vi "Measurement Logic.vi"(8 "error in":errorcluster, 10 "Measurement Context":refnum<class "MeasurementContext.lvclass">, 11 "Measurement Configuration":T2={"Load Current in A"=0.005, "Nominal Output Voltage in V"=3.3, "Start"=4.0, "Stop"=6.0, "Step"=0.1, "Input SMU"="", "Load SMU"="", "Input DMM"="", "Load DMM"=""} {"Nominal Output Voltage in V" format="%#_13g"; "Load Current in A" format="%#_13g"}) -> (0 "error out":errorcluster, 2 "Measurement Context out":refnum<class "MeasurementContext.lvclass">, 3 "Measurement Results":T1)   [LabVIEW 2020, in "LineRegulation.lvlib"]
uses:
  LineRegulation.lvlib
  Measurement Configuration.ctl
  Measurement Results.ctl
  RPC Service/MeasurementContext/MeasurementContext.lvclass
  TestInputs.ctl
  Reusables/Advanced Settings.ctl
  Reusables/Prepare Fn Configurations.ctl
  Reusables/Load Output Function.ctl
  Reusables/Stimulus And Measure.ctl
  TestResults.ctl
  334814aa-6350-40fc-9da7-130e073bd573.vi
panel:
  out "Line Regulation":cluster{"Iload (mA)":dbl[], "Vout (V)":dbl[]}(graph)
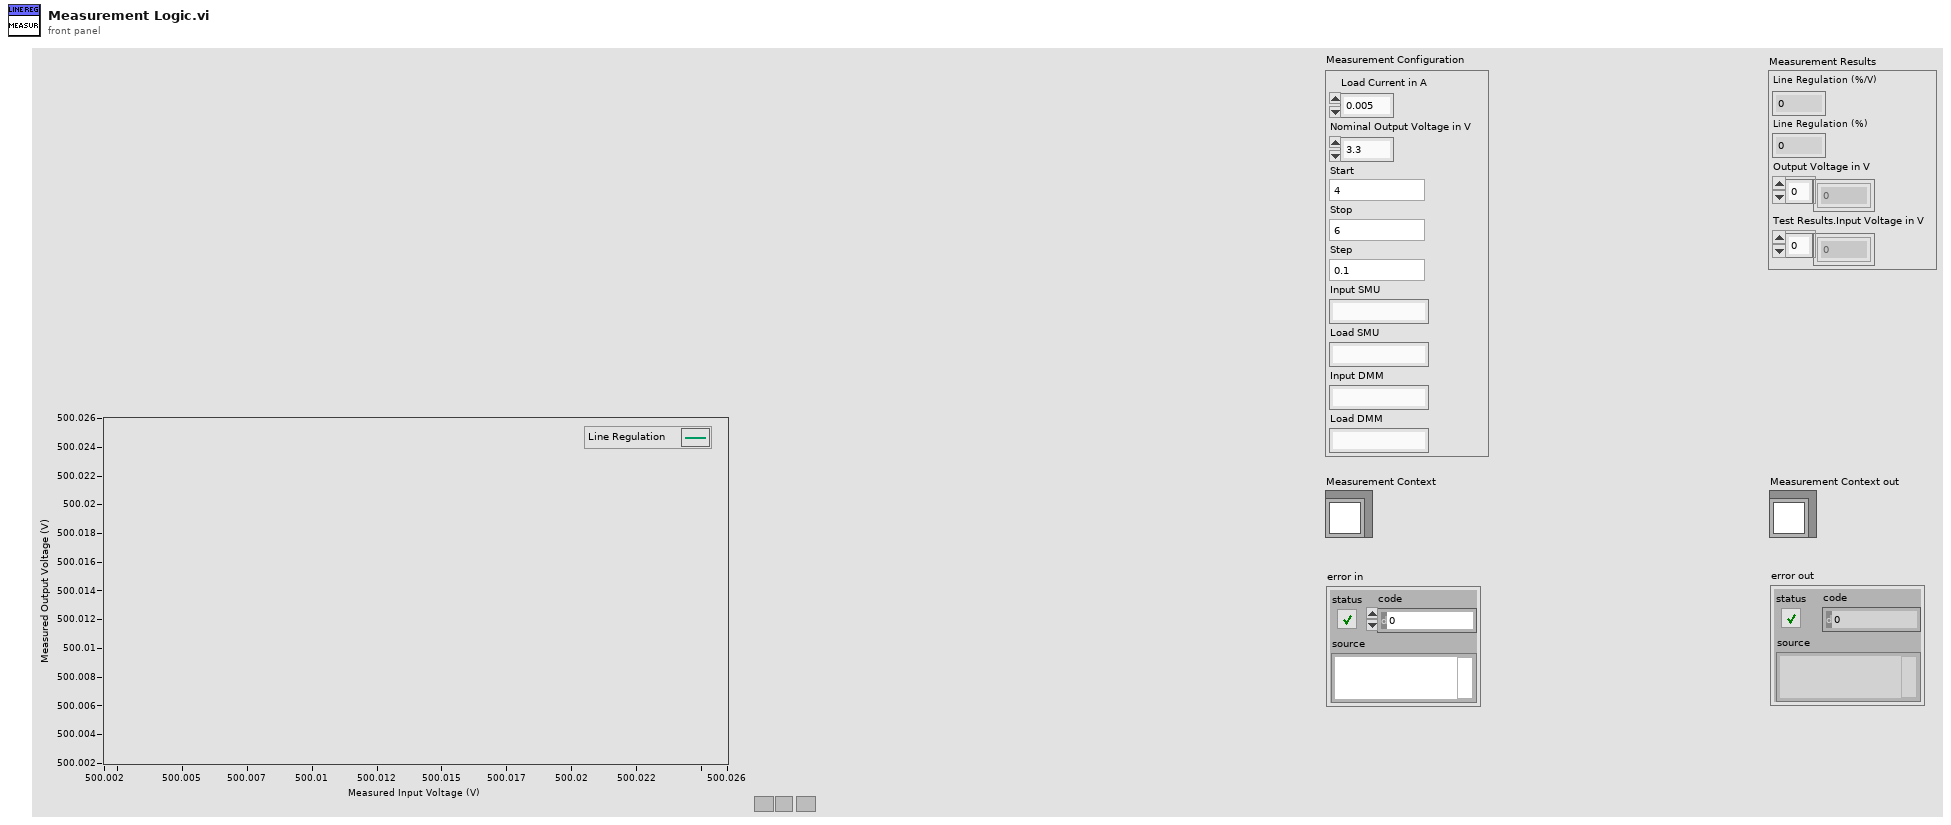
[diagram p1: front panel]
types:
  T1 = typedef "LineRegulation.lvlib/Measurement Results.ctl" = cluster{"Line Regulation (%/V)":dbl, "Line Regulation (%)":dbl, "Output Voltage in V":dbl[], "Test Results.Input Voltage in V":dbl[]}
  T2 = typedef "LineRegulation.lvlib/Measurement Configuration.ctl" = cluster{"Load Current in A":dbl, "Nominal Output Voltage in V":dbl, "Start":dbl, "Stop":dbl, "Step":dbl, "Input SMU":string, "Load SMU":string, "Input DMM":string, "Load DMM":string}
  T3 = typedef "LineRegulation.lvlib/TestInputs.ctl" = cluster{"Load Current in A":dbl, "Input Voltage in V":dbl[], "Nominal Output Voltage in V":dbl, "Advance Setting":T4}
  T4 = typedef "Advanced Settings.ctl" = cluster{"Prepare":T5, "Stimulus And Measure":T7}
  T5 = typedef "Prepare Fn Configurations.ctl" = cluster{"Load SMU Output Function":T6}
  T6 = typedef "Load Output Function.ctl" = enum16{"VoltageSource", "CurrentSource"}
  T7 = typedef "Stimulus And Measure.ctl" = cluster{"Loop Delay in milliSecond":u32}
  T8 = typedef "LineRegulation.lvlib/TestResults.ctl" = cluster{"Input Voltage in V":dbl[], "Input Current in A":dbl[], "Output Voltage in V":dbl[], "Load Current in A":dbl[], "Line Regulation in %/V":dbl, "Line Regulation in %":dbl}
  T9 = cluster{"Test Inputs":T3, "Test Results":T8, "Test Results[][]":string[][], "SMU V":refnum<k15>, "Input DMM":refnum<k15>, "Load DMM":refnum<k15>, "SMU I":refnum<k15>}
  T10 = cluster{"Input Voltage in V":dbl[], "Output Voltage in V":dbl[]}
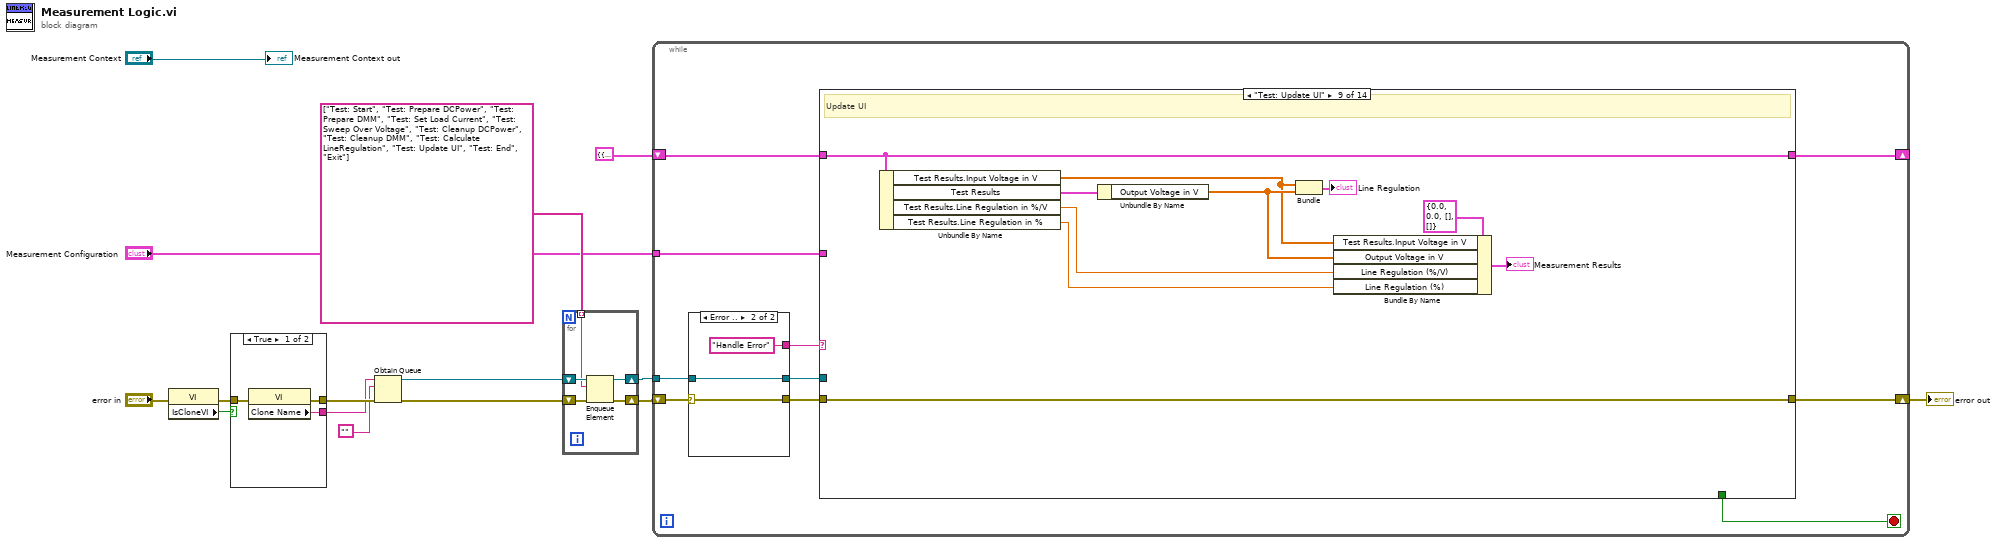
[diagram p0: block diagram]
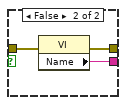
[diagram p2: hidden frame]
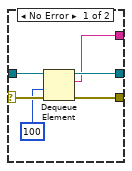
[diagram p3: hidden frame]
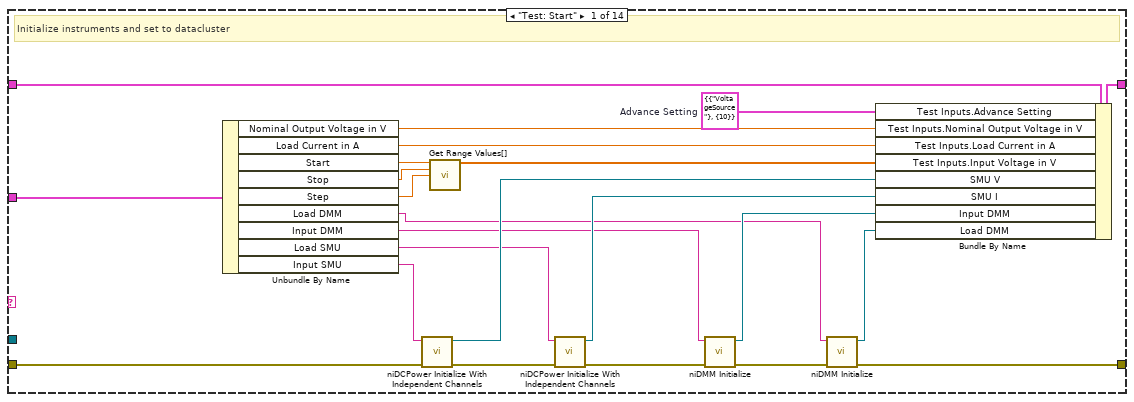
[diagram p4: hidden frame]
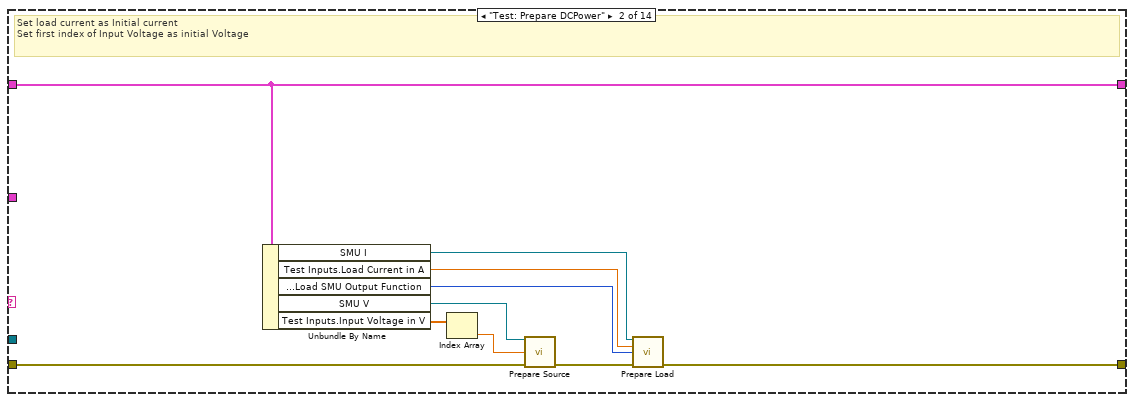
[diagram p5: hidden frame]
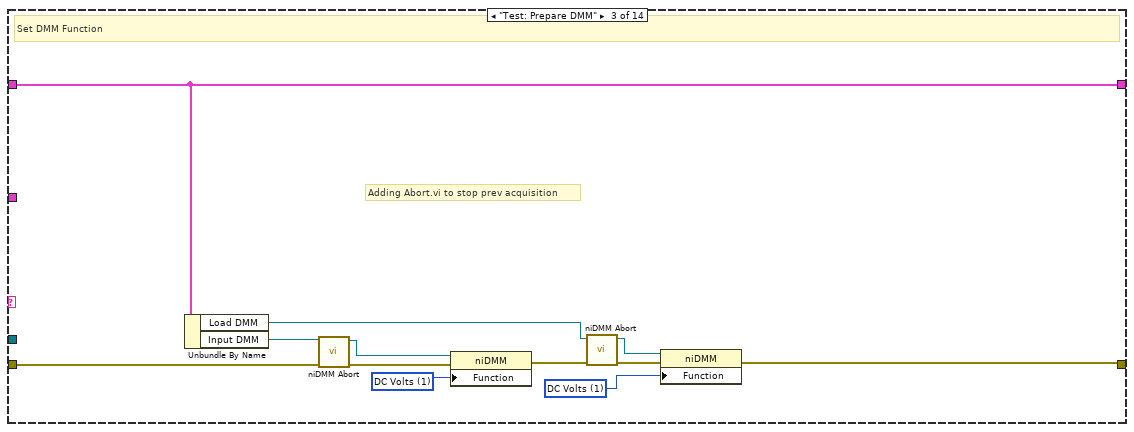
[diagram p6: hidden frame]
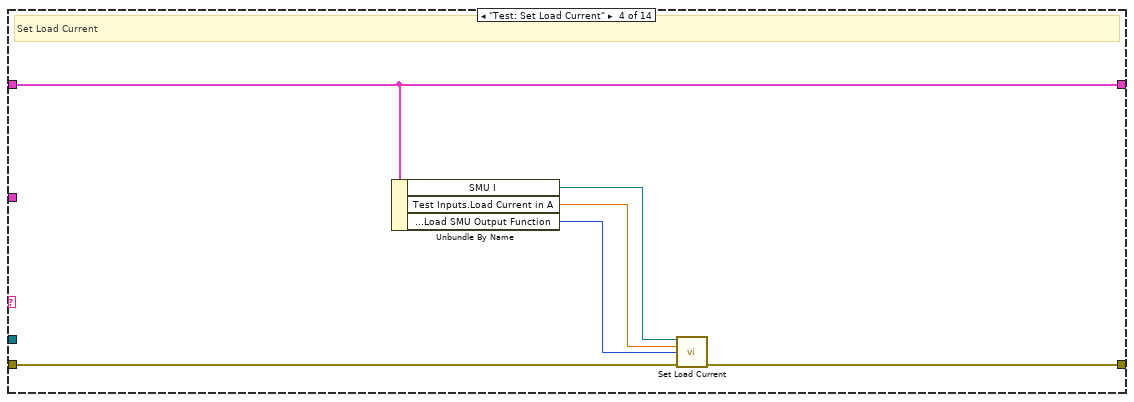
[diagram p7: hidden frame]
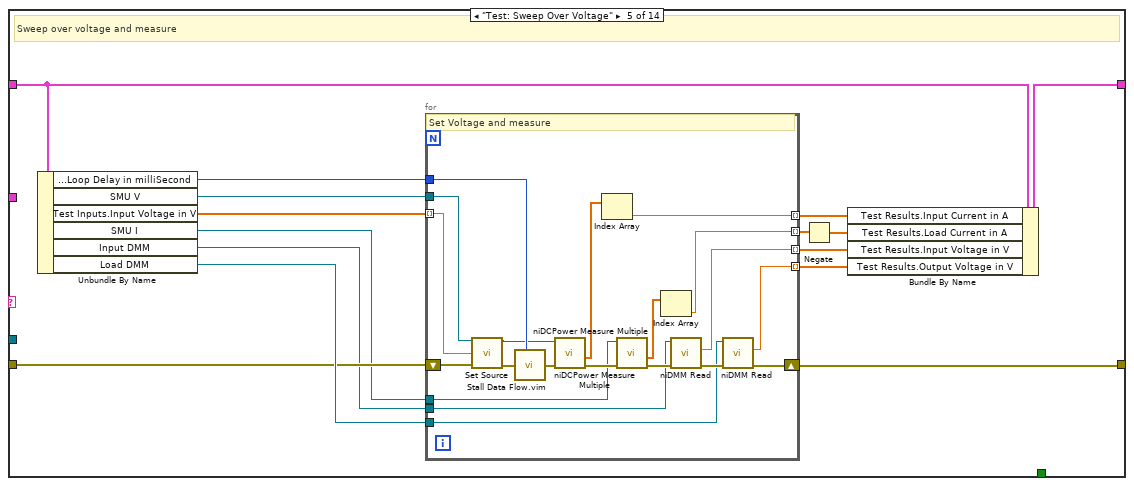
[diagram p8: hidden frame]
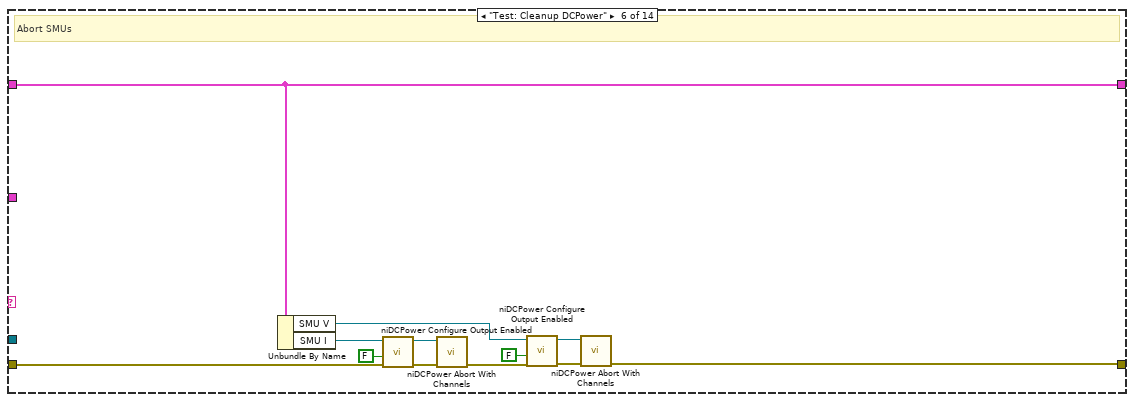
[diagram p9: hidden frame]
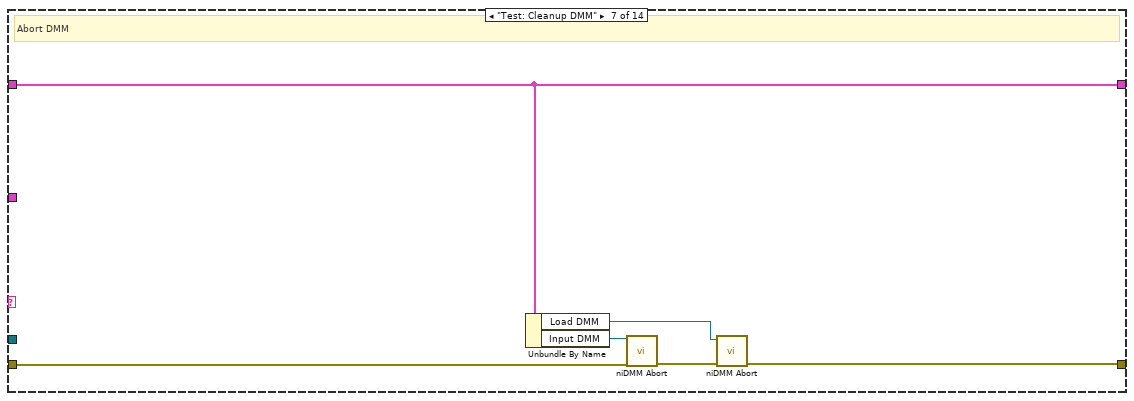
[diagram p10: hidden frame]
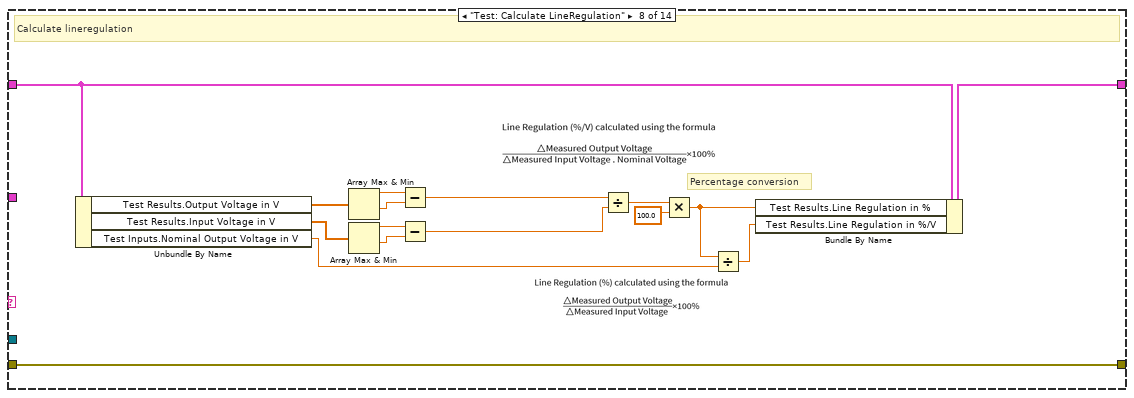
[diagram p11: hidden frame]
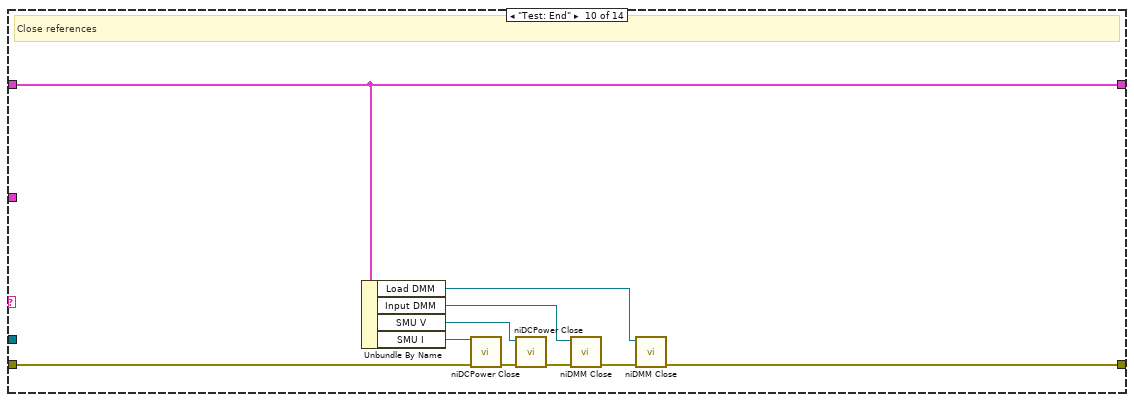
[diagram p12: hidden frame]
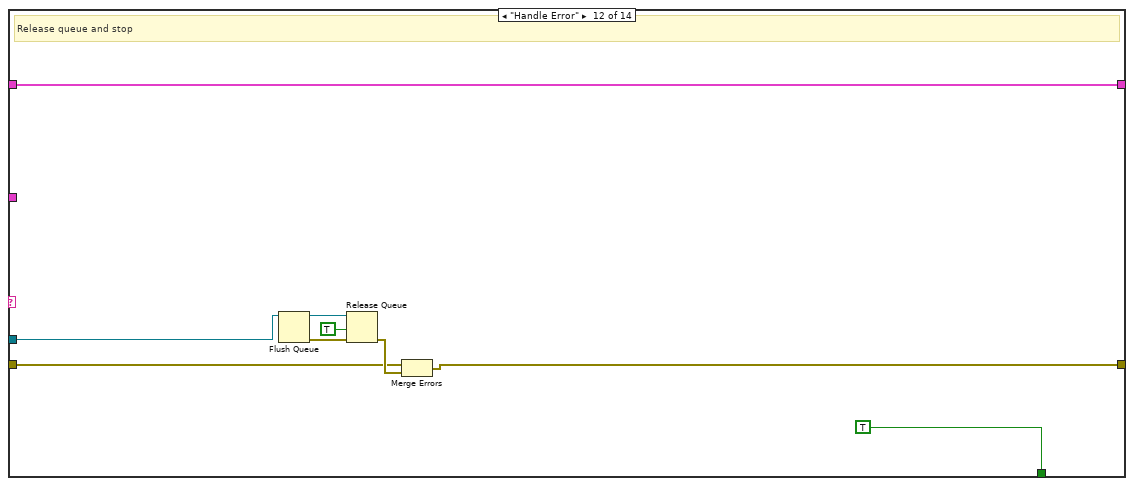
[diagram p14: hidden frame]
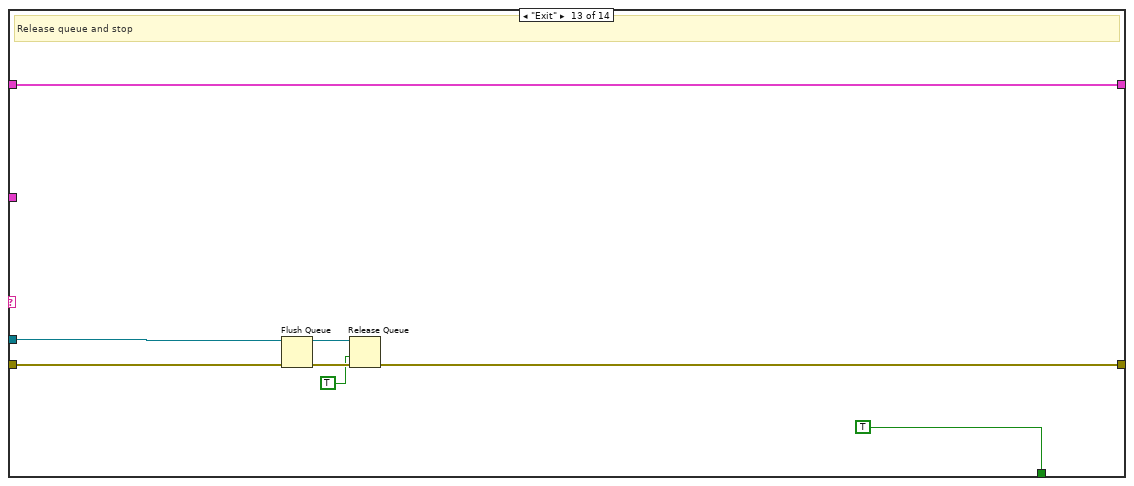
[diagram p15: hidden frame]
diagram:
  n1 = property class="VI"(error in="error in") -> (error out=w8:errorcluster, "IsCloneVI"=w9:bool)  [unwired: 1 in, 1 out]
  n2 = case shown="True" w9 {
    tunnel: [w18 w21] -> w14
    tunnel: [w17 w20] -> w13
    tunnel: w8 -> [w16 w19]
    frame True {
      n3 = property class="VI"(error in=w16) -> (error out=w18:errorcluster, "Clone Name"=w17:string)  [unwired: 1 in, 1 out]
    }
    frame False {
      n4 = property class="VI"(error in=w19) -> (error out=w21:errorcluster, "Name"=w20:string)  [unwired: 1 in, 1 out]
    }
  }
  n5 = Obtain Queue(name (unnamed)=w13, element data type="", error in (no error)=w14) -> (queue out=w11:refnum<queue>, error out=w12:errorcluster)  [unwired: 2 in, 1 out]
  n6 = for {
    shift-right: [w24] -> w7
    shift-left: w12 -> [w26]
    shift-right: [w23] -> w6
    shift-left: w11 -> [w25]
    tunnel: string[] ["Test: Start", "Test: Prepare DCPower", "Test: Prepare DMM", "Test: Set Load Current", "Test: Sweep Over Voltage", "Test: Cleanup DCPower", "Test: Cleanup DMM", "Test: Calculate LineRegulation", "Test: Update UI", "Test: End", "Exit"] -> [w22] mode=indexing
    n7 = Enqueue Element(queue=w25, element=w22, error in (no error)=w26) -> (queue out=w23:refnum<queue>, error out=w24:errorcluster)  [unwired: 1 in, 1 out]
  }
  n8 = while {
    shift-right: [w36] -> w2
    shift-left: w7 -> [w32]
    shift-right: [w34] -> _
    shift-left: T9 {"Test Inputs"={"Load Current in A"=0.0, "Input Voltage in V"=[], "Nominal Output Voltage in V"=0.0, "Advance Setting"={"Prepare"={"Load SMU Output Function"=enum."VoltageSource"}, "Stimulus And Measure"={"Loop Delay in milliSecond"=1}}}, "Test Results"={"Input Voltage in V"=[], "Input Current in A"=[], "Output Voltage in V"=[], "Load Current in A"=[], "Line Regulation in %/V"=0.0, "Line Regulation in %"=0.0}, "Test Results[][]"=[], "SMU V"="", "Input DMM"="", "Load DMM"="", "SMU I"=""} -> [w35]
    tunnel: w6 -> [w28]
    tunnel: "Measurement Configuration" -> [w27]
    stop <- w33 stop-if-true
    n9 = case shown="Error .." w32 {
      selector: w32 -> [w42 w45]
      tunnel: [w41 w45] -> w29
      tunnel: w28 -> [w40 w44]
      tunnel: [w39 w44] -> w31
      tunnel: [w38 "Handle Error"] -> w30
      frame No Error {
        n10 = Dequeue Element(queue=w40, timeout in ms (-1)=100, error in (no error)=w42) -> (queue out=w39:refnum<queue>, element=w38:string, error out=w41:errorcluster)  [unwired: 1 out]
      }
      frame Error {
      }
    }
    n11 = case shown="\"Test: Update UI\"" w30 {
      tunnel: w31 -> [_ _ _ _ _ _ _ _ _ _ _ w190 w197 _]
      tunnel: w29 -> [w51 w71 w79 w93 w99 w132 w144 w150 w168 w176 w187 w188 w199 w205]
      tunnel: [w50 w72 w81 w94 w102 w140 w147 w150 w168 w179 w187 w195 w198 w205] -> w36
      tunnel: w35 -> [w67 w77 w87 w96 w100 w139 w149 w151 w173 w185 w186 w196 w204 w206]
      tunnel: [w68 w77 w87 w96 w101 w139 w149 w152 w173 w185 w186 w196 w204 w206] -> w34
      tunnel: [_ _ _ _ _ _ _ _ _ _ _ TRUE TRUE _] -> w33
      tunnel: w27 -> [w46 _ _ _ _ _ _ _ _ _ _ _ _ _]
      frame "Test: Start" {
        w47 = T4 {"Prepare"={"Load SMU Output Function"=enum."VoltageSource"}, "Stimulus And Measure"={"Loop Delay in milliSecond"=10}}  # Advance Setting
        # "Initialize instruments and set to datacluster"
        n12 = Unbundle By Name(w46) -> ("Nominal Output Voltage in V"=w49:dbl, "Load Current in A"=w48:dbl, "Start"=w59:dbl, "Stop"=w58:dbl, "Step"=w57:dbl, "Load DMM"=w55:string, "Input DMM"=w54:string, "Load SMU"=w53:string, "Input SMU"=w52:string)
        n13 = call <instrlib>:"niDCPower Initialize With Independent Channels.vi"("error in (no error)"=w51, "resource name"=w52) -> ("error out"=w63:errorcluster, "instrument handle out"=w66:refnum<k15>)  [unwired: 8 in]
        n14 = call "Get Range Values[].vi"("Start"=w59, "Stop"=w58, "Step Size"=w57) -> ("Values[]"=w56:dbl[])  [unwired: 12 in]
        n15 = call <instrlib>:"niDCPower Initialize With Independent Channels.vi"("error in (no error)"=w63, "resource name"=w53) -> ("error out"=w62:errorcluster, "instrument handle out"=w60:refnum<k15>)  [unwired: 8 in]
        n16 = call <instrlib>:"niDMM Initialize.vi"("error in (no error)"=w62, "Instrument Descriptor"=w54) -> ("error out"=w64:errorcluster, "instrument handle out"=w61:refnum<k15>)  [unwired: 8 in]
        n17 = call <instrlib>:"niDMM Initialize.vi"("error in (no error)"=w64, "Instrument Descriptor"=w55) -> ("error out"=w50:errorcluster, "instrument handle out"=w65:refnum<k15>)  [unwired: 8 in]
        n18 = Bundle By Name(cluster=w67, "Test Inputs.Advance Setting"=w47, "Test Inputs.Nominal Output Voltage in V"=w49, "Test Inputs.Load Current in A"=w48, "Test Inputs.Input Voltage in V"=w56, "SMU V"=w66, "SMU I"=w60, "Input DMM"=w61, "Load DMM"=w65) -> (w68:T9)
      }
      frame "Test: Prepare DCPower" {
        # "Set load current as Initial current\nSet first index of Input Voltage as initial Voltage"
        n19 = Unbundle By Name(w77) -> ("SMU I"=w74:refnum<k15>, "Test Inputs.Load Current in A"=w70:dbl, "Test Inputs.Advance Setting.Prepare.Load SMU Output Function"=w69:T6, "SMU V"=w76:refnum<k15>, "Test Inputs.Input Voltage in V"=w78:dbl[])
        n20 = Index Array(array=w78) -> (element=w75:dbl)  [unwired: 1 in]
        n21 = call "Prepare Source.vi"("instrument handle"=w76, "Initial Voltage Level (V)"=w75, "error in (no error)"=w71) -> ("error out"=w73:errorcluster)  [unwired: 12 in]
        n22 = call "Prepare Load.vi"("instrument handle"=w74, "Load Current Level (A)"=w70, "Load Output Function"=w69, "error in (no error)"=w73) -> ("error out"=w72:errorcluster)  [unwired: 11 in]
      }
      frame "Test: Prepare DMM" {
        w83 = 1 items=["DC Volts"=1, "AC Volts"=2, "DC Current"=3, "AC Current"=4, "2-Wire Resistance"=5, "4-Wire Resistance"=101, "Frequency"=104, "Period"=105, "AC Volts DC Coupled"=1001, "Diode"=1002, "Waveform Voltage"=1003, "Waveform Current"=1004, "Capacitance"=1005, "Inductance"=1006, "Temperature"=108] ("Configuration:Function")
        w90 = 1 items=["DC Volts"=1, "AC Volts"=2, "DC Current"=3, "AC Current"=4, "2-Wire Resistance"=5, "4-Wire Resistance"=101, "Frequency"=104, "Period"=105, "AC Volts DC Coupled"=1001, "Diode"=1002, "Waveform Voltage"=1003, "Waveform Current"=1004, "Capacitance"=1005, "Inductance"=1006, "Temperature"=108] ("Configuration:Function")
        # "Adding Abort.vi to stop prev acquisition"
        # "Set DMM Function"
        n23 = Unbundle By Name(w87) -> ("Load DMM"=w80:refnum<k15>, "Input DMM"=w86:refnum<k15>)
        n24 = call <instrlib>:"niDMM Abort.vi"("error in (no error)"=w79, "instrument handle"=w86) -> ("error out"=w89:errorcluster, "instrument handle out"=w88:refnum<k15>)  [unwired: 8 in]
        n25 = property class="niDMM"(reference=w88, error in=w89, "Function"=w90) -> (error out=w82:errorcluster)  [unwired: 1 out]
        n26 = call <instrlib>:"niDMM Abort.vi"("error in (no error)"=w82, "instrument handle"=w80) -> ("error out"=w84:errorcluster, "instrument handle out"=w85:refnum<k15>)  [unwired: 8 in]
        n27 = property class="niDMM"(reference=w85, error in=w84, "Function"=w83) -> (error out=w81:errorcluster)  [unwired: 1 out]
      }
      frame "Test: Set Load Current" {
        # "Set Load Current"
        n28 = Unbundle By Name(w96) -> ("SMU I"=w95:refnum<k15>, "Test Inputs.Load Current in A"=w92:dbl, "Test Inputs.Advance Setting.Prepare.Load SMU Output Function"=w91:T6)
        n29 = call "Set Load Current.vi"("instrument handle in"=w95, "current level"=w92, "OutputFunction"=w91, "error in (no error)"=w93) -> ("error out"=w94:errorcluster)  [unwired: 10 in, 1 out]
      }
      frame "Test: Sweep Over Voltage" {
        # "Sweep over voltage and measure"
        n30 = Unbundle By Name(w100) -> ("Test Inputs.Advance Setting.Stimulus And Measure.Loop Delay in milliSecond"=w109:u32, "SMU V"=w111:refnum<k15>, "Test Inputs.Input Voltage in V"=w110:dbl[], "SMU I"=w97:refnum<k15>, "Input DMM"=w98:refnum<k15>, "Load DMM"=w108:refnum<k15>)
        n31 = for {
          tunnel: w111 -> [w130]
          tunnel: w110 -> [w129] mode=indexing
          tunnel: w109 -> [w127]
          tunnel: w98 -> [w120]
          tunnel: w108 -> [w119]
          tunnel: [w118] -> w106 mode=indexing
          tunnel: [w117] -> w105 mode=indexing
          tunnel: [w116] -> w104 mode=indexing
          tunnel: [w115] -> w103 mode=indexing
          shift-right: [w114] -> w102
          shift-left: w99 -> [w131]
          tunnel: w97 -> [w112]
          # "Set Voltage and measure"
          n32 = call "Set Source.vi"("instrument handle in"=w130, "Vin in V"=w129, "error in (no error)"=w131) -> ("instrument handle out"=w113:refnum<k15>, "error out"=w128:errorcluster)  [unwired: 11 in]
          n33 = call "Stall Data Flow.vim"("value in"=w128, "milliseconds to wait"=w127) -> ("value out"=w121:errorcluster)  [unwired: 1 out]
          n34 = call <instrlib>:"niDCPower Measure Multiple.vi"("error in (no error)"=w121, "instrument handle"=w113) -> ("error out"=w123:errorcluster, "current measurements"=w126:dbl[])  [unwired: 6 in, 2 out]
          n35 = Index Array(array=w126) -> (element=w118:dbl)  [unwired: 1 in]
          n36 = call <instrlib>:"niDCPower Measure Multiple.vi"("error in (no error)"=w123, "instrument handle"=w112) -> ("error out"=w122:errorcluster, "current measurements"=w124:dbl[])  [unwired: 6 in, 2 out]
          n37 = Index Array(array=w124) -> (element=w117:dbl)  [unwired: 1 in]
          n38 = call <instrlib>:"niDMM Read.vi"("error in (no error)"=w122, "instrument handle"=w120) -> ("error out"=w125:errorcluster, "Measurement"=w116:dbl)  [unwired: 7 in, 1 out]
          n39 = call <instrlib>:"niDMM Read.vi"("error in (no error)"=w125, "instrument handle"=w119) -> ("error out"=w114:errorcluster, "Measurement"=w115:dbl)  [unwired: 7 in, 1 out]
        }
        n40 = Negate(x=w105) -> (-x=w107:dbl[])
        n41 = Bundle By Name(cluster=w100, "Test Results.Input Current in A"=w106, "Test Results.Load Current in A"=w107, "Test Results.Input Voltage in V"=w104, "Test Results.Output Voltage in V"=w103) -> (w101:T9)
      }
      frame "Test: Cleanup DCPower" {
        # "Abort SMUs"
        n42 = Unbundle By Name(w139) -> ("SMU V"=w138:refnum<k15>, "SMU I"=w133:refnum<k15>)
        n43 = call <instrlib>:"niDCPower Configure Output Enabled.vi"("error in (no error)"=w132, "output enabled"=FALSE, "instrument handle"=w133) -> ("error out"=w134:errorcluster, "instrument handle out"=w137:refnum<k15>)  [unwired: 7 in]
        n44 = call <instrlib>:"niDCPower Abort With Channels.vi"("error in (no error)"=w134, "instrument handle"=w137) -> ("error out"=w135:errorcluster)  [unwired: 8 in, 1 out]
        n45 = call <instrlib>:"niDCPower Configure Output Enabled.vi"("error in (no error)"=w135, "output enabled"=FALSE, "instrument handle"=w138) -> ("error out"=w142:errorcluster, "instrument handle out"=w141:refnum<k15>)  [unwired: 7 in]
        n46 = call <instrlib>:"niDCPower Abort With Channels.vi"("error in (no error)"=w142, "instrument handle"=w141) -> ("error out"=w140:errorcluster)  [unwired: 8 in, 1 out]
      }
      frame "Test: Cleanup DMM" {
        # "Abort DMM"
        n47 = Unbundle By Name(w149) -> ("Load DMM"=w146:refnum<k15>, "Input DMM"=w145:refnum<k15>)
        n48 = call <instrlib>:"niDMM Abort.vi"("error in (no error)"=w144, "instrument handle"=w145) -> ("error out"=w148:errorcluster)  [unwired: 8 in, 1 out]
        n49 = call <instrlib>:"niDMM Abort.vi"("error in (no error)"=w148, "instrument handle"=w146) -> ("error out"=w147:errorcluster)  [unwired: 8 in, 1 out]
      }
      frame "Test: Calculate LineRegulation" {
        # "Percentage conversion"
        # "Calculate lineregulation"
        n50 = Unbundle By Name(w151) -> ("Test Results.Output Voltage in V"=w163:dbl[], "Test Results.Input Voltage in V"=w158:dbl[], "Test Inputs.Nominal Output Voltage in V"=w154:dbl)
        n51 = Array Max & Min(array=w163) -> (max value=w165:dbl, min value=w161:dbl)  [unwired: 2 out]
        n52 = Array Max & Min(array=w158) -> (max value=w159:dbl, min value=w160:dbl)  [unwired: 2 out]
        n53 = Subtract(x=w165, y=w161) -> (x-y=w162:dbl)
        n54 = Subtract(x=w159, y=w160) -> (x-y=w157:dbl)
        n55 = Divide(x=w162, y=w157) -> (x/y=w156:dbl)
        n56 = Multiply(x=w156, y=100.0) -> (x*y=w155:dbl)
        n57 = Divide(x=w155, y=w154) -> (x/y=w153:dbl)
        n58 = Bundle By Name(cluster=w151, "Test Results.Line Regulation in %"=w155, "Test Results.Line Regulation in %/V"=w153) -> (w152:T9)
      }
      frame "Test: Update UI" {
        # "Update UI"
        n59 = Unbundle By Name(w173) -> ("Test Results.Input Voltage in V"=w169:dbl[], "Test Results"=w174:T8, "Test Results.Line Regulation in %/V"=w172:dbl, "Test Results.Line Regulation in %"=w171:dbl)
        n60 = Unbundle By Name(w174) -> ("Output Voltage in V"=w170:dbl[])
        n61 = Bundle("Input Voltage in V"=w169, "Output Voltage in V"=w170) -> (→"Line Regulation":T10)  [unwired: 1 in]
        n62 = Bundle By Name(cluster=T1 {"Line Regulation (%/V)"=0.0, "Line Regulation (%)"=0.0, "Output Voltage in V"=[], "Test Results.Input Voltage in V"=[]} ("Measurement Results"), "Test Results.Input Voltage in V"=w169, "Output Voltage in V"=w170, "Line Regulation (%/V)"=w172, "Line Regulation (%)"=w171) -> (→"Measurement Results":T1)
      }
      frame "Test: End" {
        # "Close references"
        n63 = Unbundle By Name(w185) -> ("Load DMM"=w180:refnum<k15>, "Input DMM"=w181:refnum<k15>, "SMU V"=w184:refnum<k15>, "SMU I"=w178:refnum<k15>)
        n64 = call <instrlib>:"niDCPower Close.vi"("error in (no error)"=w176, "instrument handle"=w178) -> ("error out"=w177:errorcluster)  [unwired: 9 in]
        n65 = call <instrlib>:"niDCPower Close.vi"("error in (no error)"=w177, "instrument handle"=w184) -> ("error out"=w183:errorcluster)  [unwired: 9 in]
        n66 = call <instrlib>:"niDMM Close.vi"("error in (no error)"=w183, "instrument handle"=w181) -> ("error out"=w182:errorcluster)  [unwired: 9 in]
        n67 = call <instrlib>:"niDMM Close.vi"("error in (no error)"=w182, "instrument handle"=w180) -> ("error out"=w179:errorcluster)  [unwired: 9 in]
      }
      frame "----Misc------" {
      }
      frame "Handle Error" {
        # "Release queue and stop"
        n68 = Flush Queue(queue=w190) -> (queue out=w193:refnum<queue>, error out=w192:errorcluster)  [unwired: 1 in, 1 out]
        n69 = Release Queue(queue=w193, force destroy? (F)=TRUE, error in (no error)=w192) -> (error out=w189:errorcluster)  [unwired: 2 out]
        n70 = Merge Errors(w188, w189) -> (w195:errorcluster)
      }
      frame "Exit" {
        # "Release queue and stop"
        n71 = Flush Queue(queue=w197, error in (no error)=w199) -> (queue out=w202:refnum<queue>, error out=w201:errorcluster)  [unwired: 1 out]
        n72 = Release Queue(queue=w202, force destroy? (F)=TRUE, error in (no error)=w201) -> (error out=w198:errorcluster)  [unwired: 2 out]
      }
      frame "", Default {
        # "Do nothing"
      }
    }
  }
  "error out" <- w2
  "Measurement Context out" <- "Measurement Context"
